vi "PH_Stepmotor_BaseClass.Axis Information to Data String.vi"(1 "Axis Information":T1) -> (0 "Data String":string)   [LabVIEW 2014, in "PH_Stepmotor_BaseClass.lvlib"]
uses:
  PH_Stepmotor_BaseClass.lvlib
  PH_Stepmotor_BaseClass.Axis Information.ctl
  PH_Stepmotor_BaseClass.Axis Activity.ctl
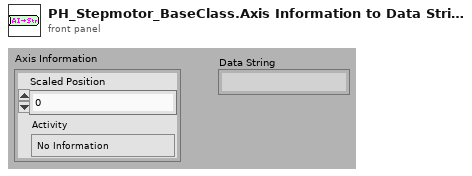
[diagram p1: front panel]
types:
  T1 = typedef "PH_Stepmotor_BaseClass.lvlib/PH_Stepmotor_BaseClass.Axis Information.ctl" = cluster{"Scaled Position":dbl, "Activity":T2}
  T2 = typedef "PH_Stepmotor_BaseClass.lvlib/PH_Stepmotor_BaseClass.Axis Activity.ctl" = enum16{"No Information", "stopped", "running", "Failure", "Alarm", "stopped at backward ES", "stopped at foreward ES"}
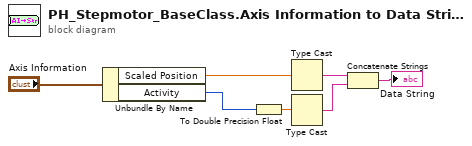
[diagram p0: block diagram]
diagram:
  n1 = Unbundle By Name("Axis Information") -> ("Scaled Position"=w2:dbl, "Activity"=w1:T2)
  n2 = To Double Precision Float(number=w1) -> (double precision float=w4:dbl)
  n3 = Type Cast(x=w2) -> (*(type *) &x=w6:string)  [unwired: 1 in]
  n4 = Type Cast(x=w4) -> (*(type *) &x=w7:string)  [unwired: 1 in]
  n5 = Concatenate Strings(w6, w7) -> (→"Data String":string)
